vi "CRYCursor InsDel.vi"(10 "Graph VI Ref":refnum<vi>, 11 "sAction":string) -> ()   [LabVIEW 2013]
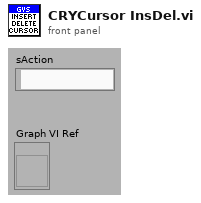
[diagram p1: front panel]
types:
  T1 = typedef "LVBoundsTypeDef.ctl" = cluster{"Width":u32, "Height":u32}
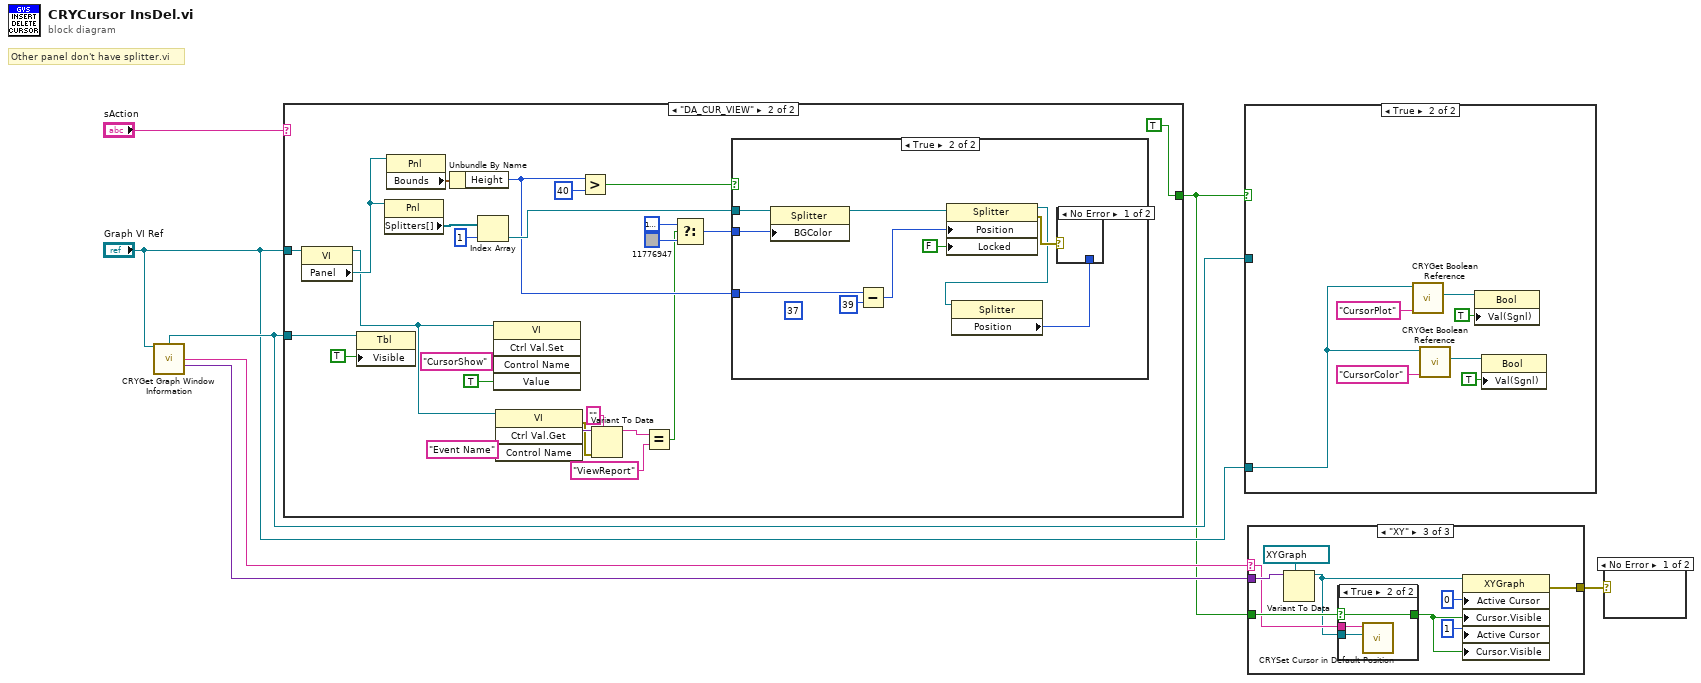
[diagram p0: block diagram]
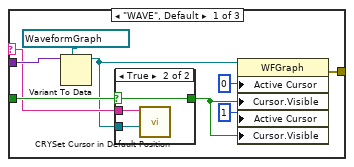
[diagram p3: hidden frame]
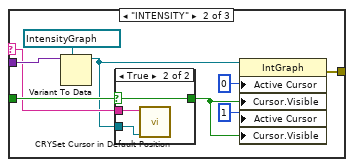
[diagram p5: hidden frame]
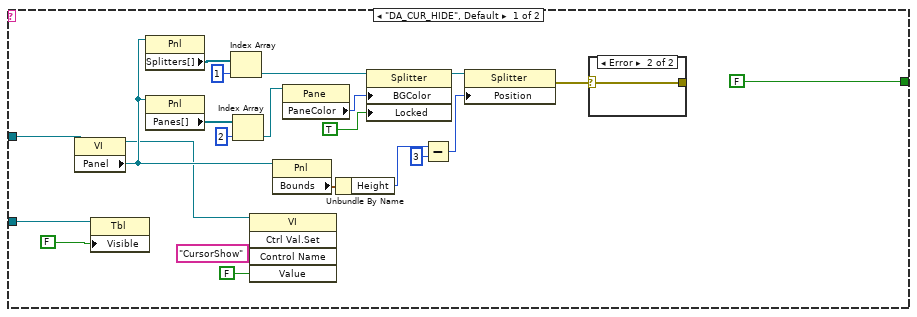
[diagram p9: hidden frame]
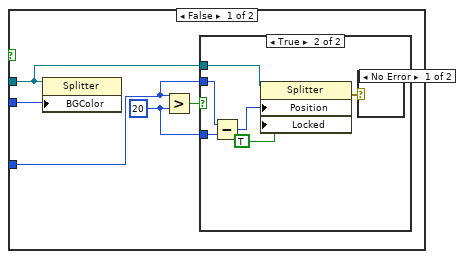
[diagram p11: hidden frame]
diagram:
  # "Other panel don't have splitter.vi"
  n1 = call "CRYGet Graph Window Information.vi"("pGraph VI In"="Graph VI Ref") -> ("Cursor Ref Out"=w6:refnum<vi>, "Graph Type Out"=w4:string, "Graph Control Ref Out"=w3:variant)  [unwired: 4 in, 8 out]
  n2 = case shown="\"DA_CUR_VIEW\"" "sAction" {
    tunnel: "Graph VI Ref" -> [w12 w52]
    tunnel: w6 -> [w28 w47]
    tunnel: [FALSE TRUE] -> w2
    frame "DA_CUR_HIDE", Default {
      n3 = property class="VI"(reference=w12) -> (reference out=w9:refnum<vi>, "Panel"=w22:refnum<vi>)  [unwired: 1 in, 1 out]
      n4 = property class="Tbl"(reference=w28, "Visible"=FALSE) -> ()  [unwired: 1 in, 2 out]
      n5 = property class="Pnl"(reference=w22) -> ("Splitters[]"=w15:refnum<vi>[])  [unwired: 1 in, 2 out]
      n6 = property class="Pnl"(reference=w22) -> ("Panes[]"=w13:refnum<vi>[])  [unwired: 1 in, 2 out]
      n7 = Index Array(array=w15, index=1) -> (element=w16:refnum<vi>)
      n8 = Index Array(array=w13, index=2) -> (element=w19:refnum<vi>)
      n9 = invoke class="VI" method="Ctrl Val.Set"(reference=w9, "Control Name"="CursorShow", "Value"=FALSE ("Visible")) -> ()  [unwired: 2 in, 5 out]
      n10 = property class="Pnl"(reference=w22) -> ("Bounds"=w23:T1)  [unwired: 1 in, 2 out]
      n11 = property class="Pane"(reference=w19) -> ("PaneColor"=w17:u32)  [unwired: 1 in, 2 out]
      n12 = Unbundle By Name(w23) -> ("Height"=w24:u32)
      n13 = property on="Property Node" class="Splitter"(reference=w16, "BGColor"=w17, "Locked"=TRUE ("Splitter Position Locked")) -> (reference out=w20:refnum<vi>)  [unwired: 1 in, 1 out]
      n14 = Subtract(x=w24, y=u32 3) -> (x-y=w26:u32)
      n15 = property on="Property Node" class="Splitter"(reference=w20, "Position"=w26) -> (error out=w21:errorcluster)  [unwired: 1 in, 1 out]
      n16 = case shown="Error" w21 {
        selector: w21 -> [w30 w31]
        tunnel: [w30 w31] -> _
        frame No Error {
        }
        frame Error {
        }
      }
    }
    frame "DA_CUR_VIEW" {
      n17 = property class="VI"(reference=w52) -> (reference out=w36:refnum<vi>, "Panel"=w54:refnum<vi>)  [unwired: 1 in, 1 out]
      n18 = property class="Tbl"(reference=w47, "Visible"=TRUE) -> ()  [unwired: 1 in, 2 out]
      n19 = property class="Pnl"(reference=w54) -> ("Splitters[]"=w56:refnum<vi>[])  [unwired: 1 in, 2 out]
      n20 = property class="Pnl"(reference=w54) -> ("Bounds"=w53:T1)  [unwired: 1 in, 2 out]
      n21 = Unbundle By Name(w53) -> ("Height"=w48:u32)
      n22 = Index Array(array=w56, index=1) -> (element=w49:refnum<vi>)
      n23 = invoke class="VI" method="Ctrl Val.Set"(reference=w36, "Control Name"="CursorShow", "Value"=TRUE ("Visible")) -> ()  [unwired: 2 in, 5 out]
      n24 = invoke class="VI" method="Ctrl Val.Get"(reference=w36, "Control Name"="Event Name") -> (error out=w39:errorcluster, "Get Control Value Variant"=w40:variant)  [unwired: 2 in, 2 out]
      n25 = Greater?(x=w48, y=u32 40) -> (0:w50:bool)
      n26 = Variant To Data(error in=w39, type="" ("Control Name"), Variant=w40) -> (data=w41:string)  [unwired: 1 out]
      n27 = Equal?(x=w41, y="ViewReport" ("Control Name")) -> (x = y?=w32:bool)
      n28 = Select(t=u32 16777226, s=w32, f=u32 11776947) -> (s? t:f=w33:u32)
      n29 = case shown="True" w50 {
        tunnel: w49 -> [w59 w76]
        tunnel: w33 -> [w61 w77]
        tunnel: w48 -> [w58 w74]
        frame False {
          w57 = u32 20 ("y")
          n30 = property on="Property Node" class="Splitter"(reference=w59, "BGColor"=w61) -> ()  [unwired: 1 in, 2 out]
          n31 = Greater?(x=w58, y=w57) -> (0:w60:bool)
          n32 = case shown="True" w60 {
            tunnel: w59 -> [_ w67]
            tunnel: w58 -> [_ w66]
            tunnel: w57 -> [_ w64]
            frame False {
            }
            frame True {
              n33 = Subtract(x=w66, y=w64) -> (x-y=w65:u32)
              n34 = property on="Property Node" class="Splitter"(reference=w67, "Position"=w65, "Locked"=TRUE ("Splitter Position Locked")) -> (error out=w63:errorcluster)  [unwired: 1 in, 1 out]
              n35 = case shown="No Error" w63 {
                frame No Error {
                }
                frame Error {
                }
              }
            }
          }
        }
        frame True {
          (unwired) u32 37 ("y")
          n36 = property on="Property Node" class="Splitter"(reference=w76, "BGColor"=w77) -> (reference out=w73:refnum<vi>)  [unwired: 1 in, 1 out]
          n37 = Subtract(x=w74, y=u32 39) -> (x-y=w71:u32)
          n38 = property on="Property Node" class="Splitter"(reference=w73, "Position"=w71, "Locked"=FALSE ("Splitter Position Locked")) -> (reference out=w69:refnum<vi>, error out=w72:errorcluster)  [unwired: 1 in]
          n39 = property on="Property Node" class="Splitter"(reference=w69) -> ("Position"=w68:i32)  [unwired: 1 in, 2 out]
          n40 = case shown="No Error" w72 {
            tunnel: w68 -> [_ _]
            frame No Error {
            }
            frame Error {
            }
          }
        }
      }
    }
  }
  n41 = case shown="True" w2 {
    tunnel: w6 -> [_ _]
    tunnel: "Graph VI Ref" -> [_ w84]
    frame False {
    }
    frame True {
      n42 = call "CRYGet Boolean Reference.vi"("Label Name"="CursorPlot" ("Control Name"), "VI Refnum"=w84) -> ("Boolean Ref"=w82:refnum<vi>)  [unwired: 7 in, 2 out]
      n43 = call "CRYGet Boolean Reference.vi"("Label Name"="CursorColor" ("Control Name"), "VI Refnum"=w84) -> ("Boolean Ref"=w79:refnum<vi>)  [unwired: 7 in, 2 out]
      n44 = property class="Bool"(reference=w82, "Val(Sgnl)"=TRUE) -> ()  [unwired: 1 in, 2 out]
      n45 = property class="Bool"(reference=w79, "Val(Sgnl)"=TRUE) -> ()  [unwired: 1 in, 2 out]
    }
  }
  n46 = case shown="\"XY\"" w4 {
    selector: w4 -> [w87 w100 w113]
    tunnel: w3 -> [w92 w105 w118]
    tunnel: w2 -> [w89 w102 w115]
    tunnel: [w85 w98 w111] -> w1
    frame "WAVE", Default {
      n47 = Variant To Data(type=refnum<vi> refnum ("XY Graph"), Variant=w92) -> (data=w86:refnum<vi>)  [unwired: 1 in, 1 out]
      n48 = case shown="True" w89 {
        selector: w89 -> [w94 w97]
        tunnel: [w94 w97] -> w88
        tunnel: w87 -> [_ w96]
        tunnel: w86 -> [_ w95]
        frame False {
        }
        frame True {
          n49 = call "CRYSet Cursor in Default Position.vi"("Wave Graph Ref"=w95, "Graph Type"=w96) -> ()  [unwired: 10 in]
        }
      }
      n50 = property on="Property Node" class="WFGraph"(reference=w86, "Active Cursor"=u32 0, "Cursor.Visible"=w88, "Active Cursor"=u32 1, "Cursor.Visible"=w88) -> (error out=w85:errorcluster)  [unwired: 1 in, 1 out]
    }
    frame "INTENSITY" {
      n51 = Variant To Data(type=refnum<vi> refnum ("XY Graph"), Variant=w105) -> (data=w99:refnum<vi>)  [unwired: 1 in, 1 out]
      n52 = case shown="True" w102 {
        selector: w102 -> [w107 w110]
        tunnel: [w107 w110] -> w101
        tunnel: w100 -> [_ w109]
        tunnel: w99 -> [_ w108]
        frame False {
        }
        frame True {
          n53 = call "CRYSet Cursor in Default Position.vi"("Intensity Graph Ref"=w108, "Graph Type"=w109) -> ()  [unwired: 10 in]
        }
      }
      n54 = property on="Property Node" class="IntGraph"(reference=w99, "Active Cursor"=u32 0, "Cursor.Visible"=w101, "Active Cursor"=u32 1, "Cursor.Visible"=w101) -> (error out=w98:errorcluster)  [unwired: 1 in, 1 out]
    }
    frame "XY" {
      n55 = Variant To Data(type=refnum<vi> refnum ("XY Graph"), Variant=w118) -> (data=w112:refnum<vi>)  [unwired: 1 in, 1 out]
      n56 = case shown="True" w115 {
        selector: w115 -> [w120 w123]
        tunnel: [w120 w123] -> w114
        tunnel: w113 -> [_ w122]
        tunnel: w112 -> [_ w121]
        frame False {
        }
        frame True {
          n57 = call "CRYSet Cursor in Default Position.vi"("XY Graph Ref"=w121, "Graph Type"=w122) -> ()  [unwired: 10 in]
        }
      }
      n58 = property on="Property Node" class="XYGraph"(reference=w112, "Active Cursor"=u32 0, "Cursor.Visible"=w114, "Active Cursor"=u32 1, "Cursor.Visible"=w114) -> (error out=w111:errorcluster)  [unwired: 1 in, 1 out]
    }
  }
  n59 = case shown="No Error" w1 {
    frame No Error {
    }
    frame Error {
    }
  }
